vi "UMLEditor_FixXmlString.vi"(8 "error in (no error)":errorcluster, 10 "XML String":string, 11 "CurrentCluster":variant) -> (0 "error out":errorcluster, 2 "XML String":string)   [LabVIEW 2016]
panel:
  out "xml string 3":string
  out "concatenated string":string
  out "substring":string
  out "Array 4":i32[](array[numeric])
  out "Array 3":i32[](array[numeric])
  out "New 2":T1
  out "xml string 2":string
  out "xml string":string
  in  "New":T1
  in  "Old":cluster{"Numeric":dbl, "Boolean":bool}
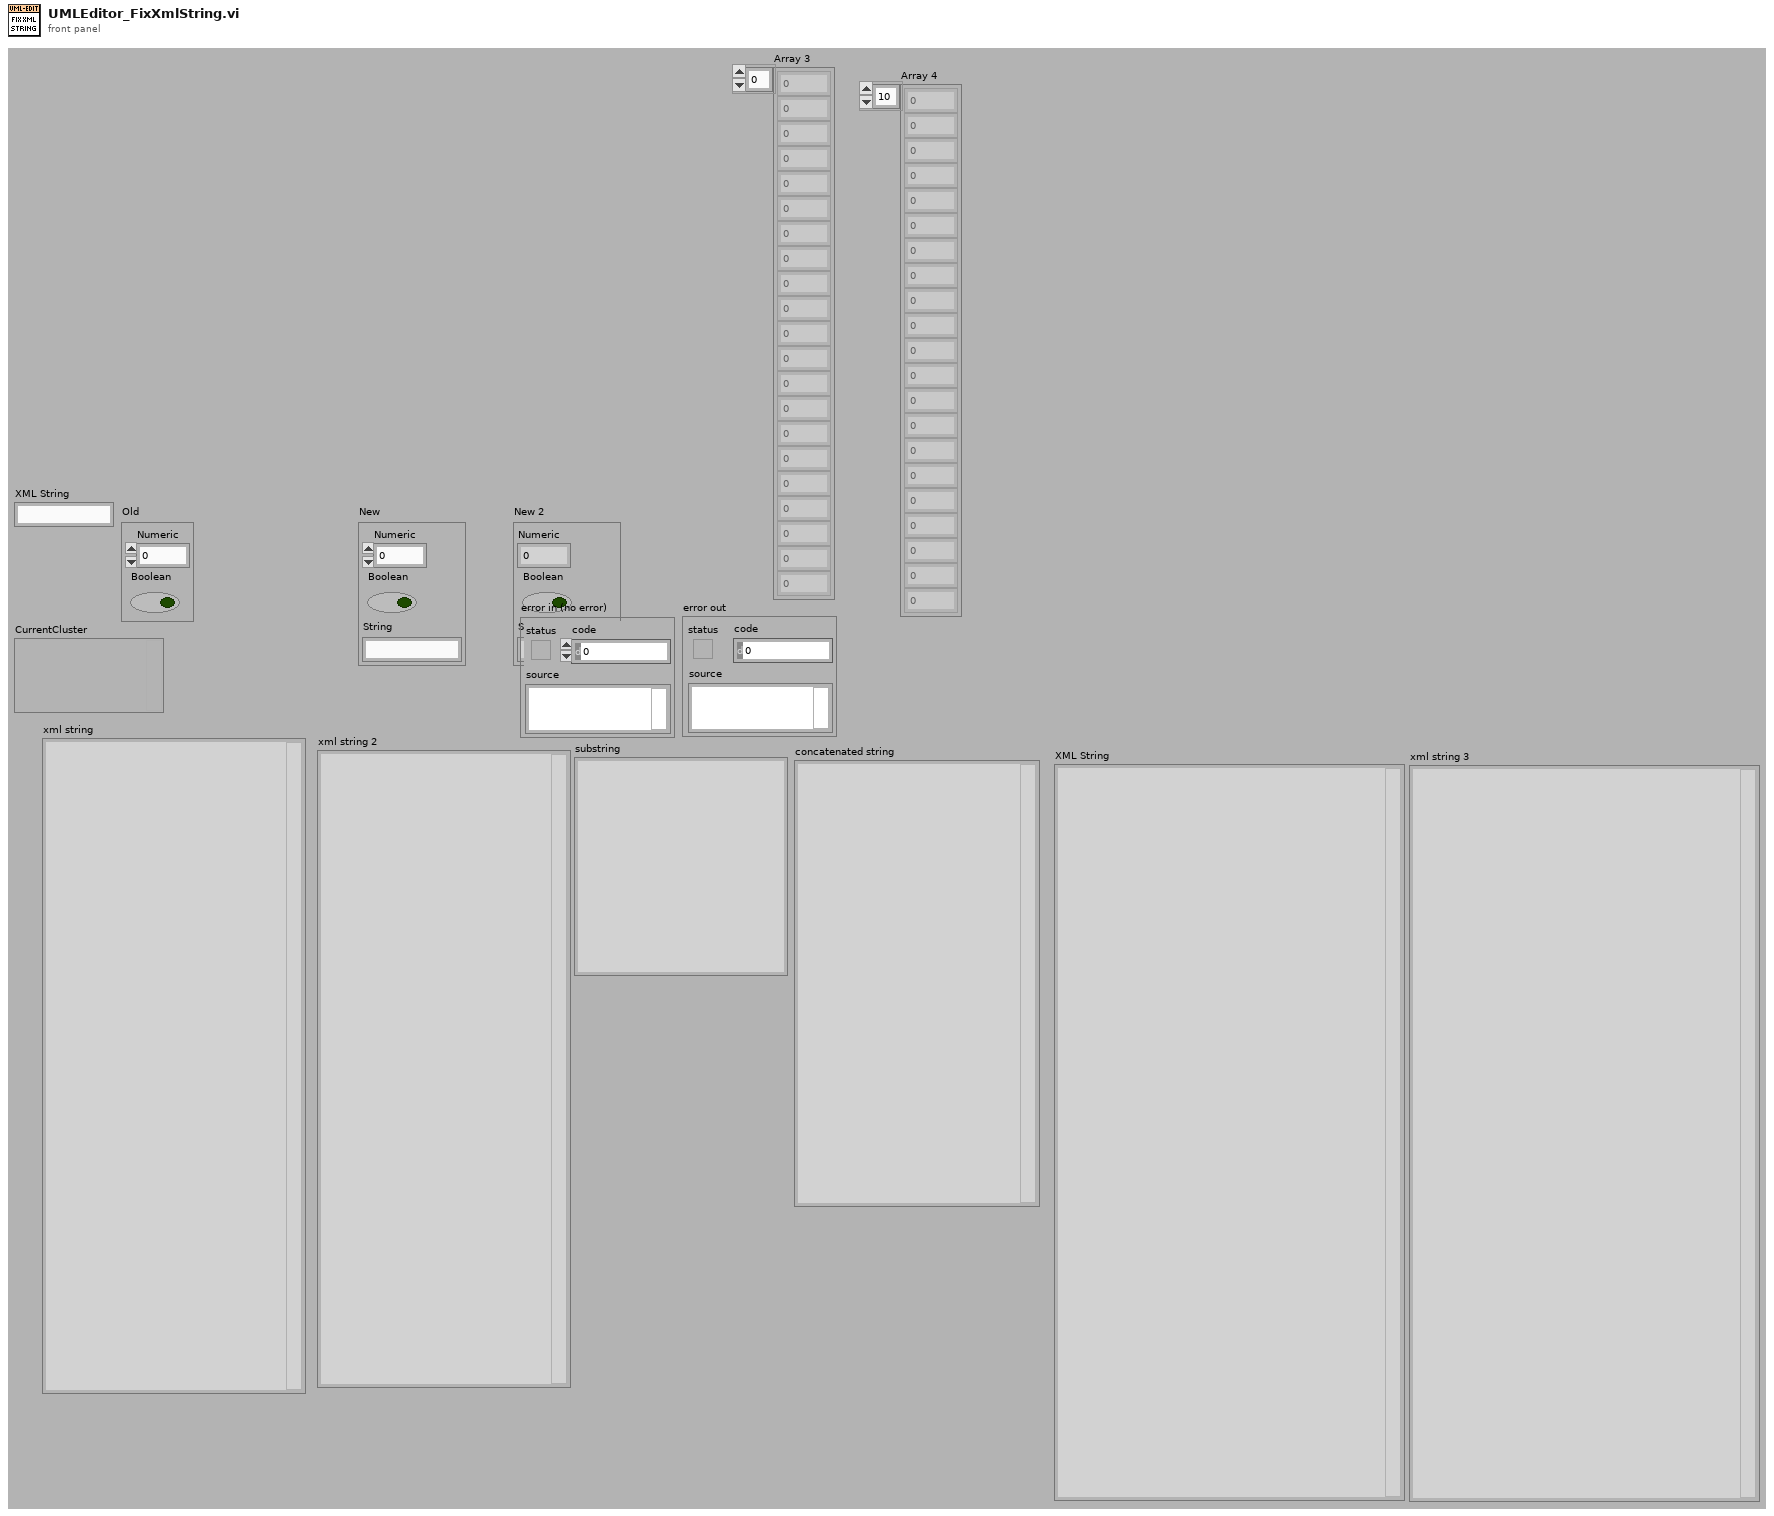
[diagram p1: front panel]
types:
  T1 = cluster{"Numeric":dbl, "Boolean":bool, "String":string}
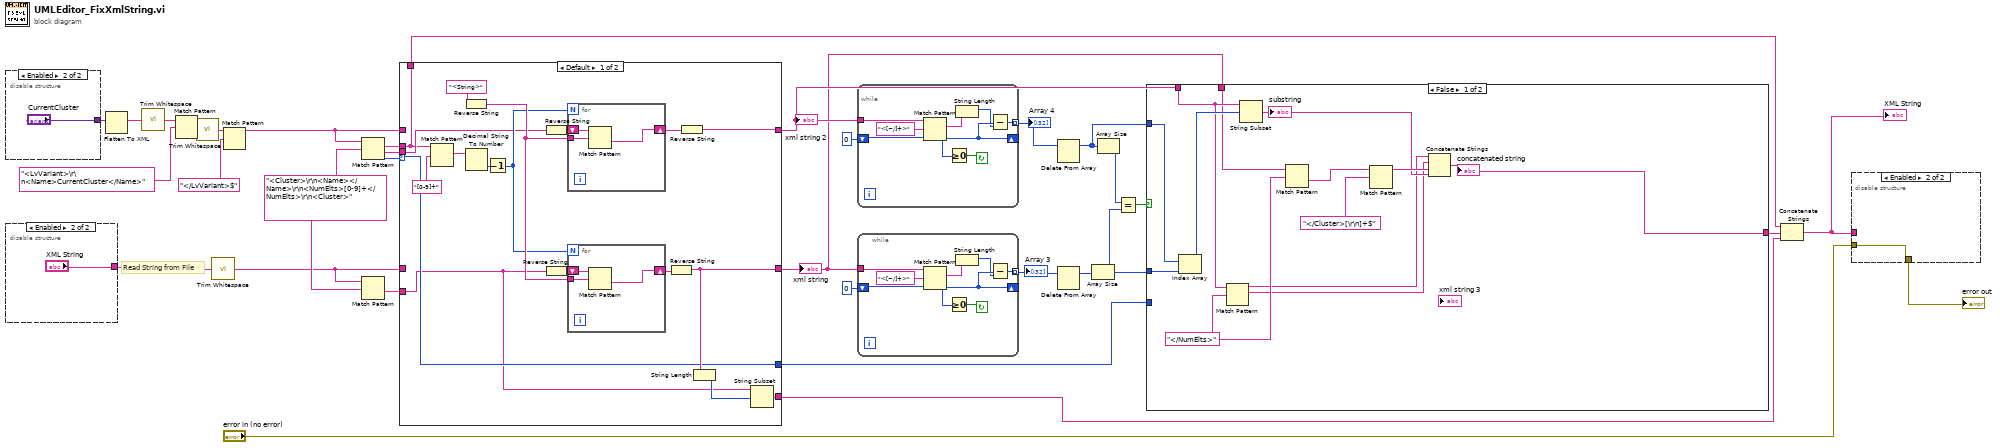
[diagram p0: block diagram]
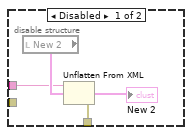
[diagram p3: hidden frame]
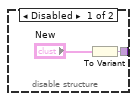
[diagram p4: hidden frame]
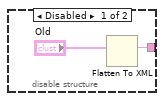
[diagram p5: hidden frame]
diagram:
  w14 = "<Cluster>\r\n<Name></Name>\r\n<NumElts>[0-9]+</NumElts>\r\n<Cluster>" ("regular expression")
  # "Read String from File"
  n1 = disable-structure shown="Enabled" {
    disable-tunnel: [w34 "CurrentCluster"] -> w21
    frame Disabled {
      n2 = To Variant(anything="New") -> (Variant=w34:variant)
    }
    frame Enabled {
    }
  }
  n3 = disable-structure shown="Enabled" {
    disable-tunnel: [w37 "XML String"] -> w23
    frame Disabled {
      n4 = Flatten To XML(anything="Old") -> (xml string=w37:string)
    }
    frame Enabled {
    }
  }
  n5 = Flatten To XML(anything=w21) -> (xml string=w25:string)
  n6 = call <vilib>:"Trim Whitespace.vi"("string"=w25) -> ("trimmed string"=w20:string)  [unwired: 1 in]
  n7 = Match Pattern(string=w20, regular expression="<LvVariant>\r\n<Name>CurrentCluster</Name>") -> (after substring=w18:string)  [unwired: 1 in, 3 out]
  n8 = call <vilib>:"Trim Whitespace.vi"("string"=w18) -> ("trimmed string"=w16:string)  [unwired: 1 in]
  n9 = call <vilib>:"Trim Whitespace.vi"("string"=w23) -> ("trimmed string"=w9:string)  [unwired: 1 in]
  n10 = Match Pattern(string=w16, regular expression="</LvVariant>$") -> (before substring=w11:string)  [unwired: 1 in, 3 out]
  n11 = Match Pattern(string=w11, regular expression=w14) -> (match substring=w13:string, after substring=w3:string, offset past match=w12:i32)  [unwired: 1 in, 1 out]
  n12 = Match Pattern(string=w9, regular expression=w14) -> (after substring=w2:string)  [unwired: 1 in, 3 out]
  n13 = case shown="Default" w12 {
    selector: w12 -> [w43 _]
    tunnel: w13 -> [w40 _]
    tunnel: w11 -> [_ w65]
    tunnel: [w51 w65] -> w10
    tunnel: w9 -> [_ w64]
    tunnel: [w46 w64] -> w8
    tunnel: [w45 _] -> w6
    tunnel: [w43 _] -> w4
    tunnel: w3 -> [w42 _]
    tunnel: w2 -> [w41 _]
    tunnel: [w40 _] -> w1
    frame Default {
      n14 = Match Pattern(string=w40, regular expression="[0-9]+") -> (match substring=w54:string)  [unwired: 1 in, 3 out]
      n15 = Reverse String(1:"<String>" ("regular expression")) -> (0:w48:string)
      n16 = Decimal String To Number(string=w54) -> (number=w53:i32)  [unwired: 2 in, 1 out]
      n17 = Decrement(x=w53) -> (x-1=w47:i32)
      n18 = Reverse String(1:w42) -> (0:w55:string)
      n19 = Reverse String(1:w41) -> (0:w49:string)
      n20 = for {
        N: w47 -> [_]
        shift-right: [w62] -> w52
        shift-left: w55 -> [w63]
        tunnel: w48 -> [w61]
        n21 = Match Pattern(string=w63, regular expression=w61) -> (after substring=w62:string)  [unwired: 1 in, 3 out]
      }
      n22 = for {
        N: w47 -> [_]
        shift-right: [w59] -> w50
        shift-left: w49 -> [w60]
        tunnel: w48 -> [w58]
        n23 = Match Pattern(string=w60, regular expression=w58) -> (after substring=w59:string)  [unwired: 1 in, 3 out]
      }
      n24 = Reverse String(1:w50) -> (0:w46:string)
      n25 = Reverse String(1:w52) -> (0:w51:string)
      n26 = String Length(string=w46) -> (length=w44:i32)
      n27 = String Subset(string=w41, offset (0)=w44) -> (substring=w45:string)  [unwired: 1 in]
    }
    frame -1 {
    }
  }
  "xml string" <- w8
  "xml string 2" <- w10
  n28 = while {
    tunnel: w10 -> [w73]
    shift-right: [w68] -> _
    shift-left: 0 ("offset past match") -> [w71]
    tunnel: [w66] -> w32 mode=indexing
    stop <- w70 continue-if-true
    n29 = Match Pattern(string=w73, regular expression="<[~/]+>", offset (0)=w71) -> (match substring=w69:string, offset past match=w68:i32)  [unwired: 2 out]
    n30 = Greater Or Equal To 0?(x=w68) -> (x >= 0?=w70:bool)
    n31 = String Length(string=w69) -> (length=w67:i32)
    n32 = Subtract(x=w68, y=w67) -> (x-y=w66:i32)
  }
  "Array 4" <- w32
  n33 = while {
    tunnel: w8 -> [w81]
    shift-right: [w76] -> _
    shift-left: 0 ("offset past match") -> [w79]
    tunnel: [w74] -> w22 mode=indexing
    stop <- w78 continue-if-true
    n34 = Match Pattern(string=w81, regular expression="<[~/]+>", offset (0)=w79) -> (match substring=w77:string, offset past match=w76:i32)  [unwired: 2 out]
    n35 = Greater Or Equal To 0?(x=w76) -> (x >= 0?=w78:bool)
    n36 = String Length(string=w77) -> (length=w75:i32)
    n37 = Subtract(x=w76, y=w75) -> (x-y=w74:i32)
  }
  "Array 3" <- w22
  n38 = Delete From Array(array=w32) -> (array with subset deleted=w26:i32[])  [unwired: 2 in, 1 out]
  n39 = Delete From Array(array=w22) -> (array with subset deleted=w31:i32[])  [unwired: 2 in, 1 out]
  n40 = Array Size(array=w31) -> (size(s)=w27:i32)
  n41 = Array Size(array=w26) -> (size(s)=w30:i32)
  n42 = Equal?(x=w30, y=w27) -> (x = y?=w28:bool)
  n43 = case shown="False" w28 {
    tunnel: [w88 w95] -> w7
    tunnel: w8 -> [w86 w95]
    tunnel: w27 -> [w94 _]
    tunnel: w26 -> [w93 _]
    tunnel: w10 -> [w87 _]
    tunnel: w4 -> [_ _]
    frame False {
      w84 = "</NumElts>" ("regular expression")
      n44 = Index Array(array=w93, index=w94) -> (element=w92:i32)
      n45 = Match Pattern(string=w87, regular expression=w84) -> (before substring=w82:string, match substring=w83:string)  [unwired: 1 in, 2 out]
      n46 = String Subset(string=w87, offset (0)=w92) -> (substring=w89:string)  [unwired: 1 in]
      "substring" <- w89
      n47 = Match Pattern(string=w86, regular expression=w84) -> (after substring=w85:string)  [unwired: 1 in, 3 out]
      n48 = Match Pattern(string=w85, regular expression="</Cluster>[\r\n]+$") -> (before substring=w90:string)  [unwired: 1 in, 3 out]
      n49 = Concatenate Strings(w82, w83, w90, w89) -> (w88:string)
      "concatenated string" <- w88
    }
    frame True {
    }
  }
  n50 = Concatenate Strings(w1, w7, w6) -> (w5:string)
  "XML String" <- w5
  n51 = disable-structure shown="Enabled" {
    disable-tunnel: [w99 w100] -> w29
    disable-tunnel: w5 -> [w96 _]
    disable-tunnel: "error in (no error)" -> [_ w100]
    frame Disabled {
      n52 = local read "New 2"() -> (w98:T1)
      n53 = Unflatten From XML(xml string=w96, type=w98) -> (value=→"New 2":T1, error out=w99:errorcluster)  [unwired: 1 in]
    }
    frame Enabled {
    }
  }
  "error out" <- w29
